vi "SC10_set_mode2.vi"(6 "error in (no error)":errorcluster, 8 "mode":i32(ring)=3 items=["manual"=1, "auto"=2, "single"=3, "repeat"=4, "external gate"=5], 9 "VISA resource name":refnum<visa-resource-name>) -> (0 "error out":errorcluster, 3 "VISA resource name out":refnum<visa-resource-name>)   [LabVIEW 2010]
panel:
  out "substring":string
  out "read buffer":string
  out "return count 3":u32
  out "return count":u32
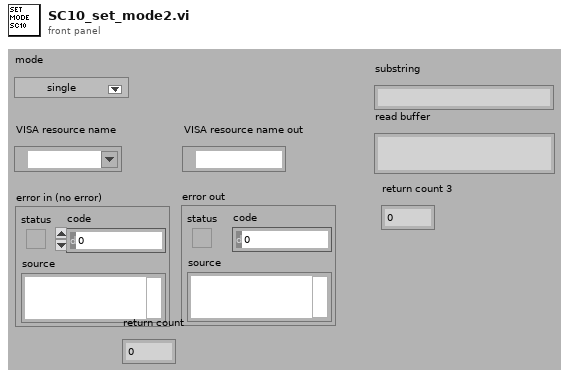
[diagram p1: front panel]
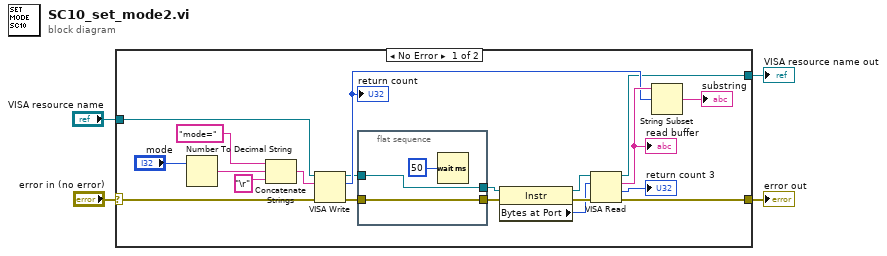
[diagram p0: block diagram]
diagram:
  n1 = case shown="No Error" "error in (no error)" {
    selector: "error in (no error)" -> [w24 w28]
    tunnel: [w6 w28] -> w3
    tunnel: [w5 w29] -> w2
    tunnel: "VISA resource name" -> [w23 w29]
    frame No Error {
      n2 = Number To Decimal String(number="mode") -> (decimal integer string=w19:string)  [unwired: 1 in]
      n3 = Concatenate Strings("mode=" ("string"), w19, "\r" ("write buffer")) -> (w20:string)
      n4 = VISA Write(VISA resource name=w23, write buffer=w20, error in (no error)=w24) -> (VISA resource name out=w8:refnum<visa-resource-name>, return count=w9:u32, error out=w7:errorcluster)
      "return count" <- w9
      n5 = flat-sequence {
        tunnel: w8 -> [w26]
        tunnel: [w26] -> w12
        tunnel: w7 -> [w25]
        tunnel: [w25] -> w13
        frame #0 {
          n6 = Wait (ms)(milliseconds to wait=u32 50) -> ()  [unwired: 1 out]
        }
      }
      n7 = property class="Instr"(reference=w12, error in=w13) -> (reference out=w11:refnum<visa-resource-name>, error out=w14:errorcluster, "Bytes at Port"=w10:u32)
      n8 = VISA Read(VISA resource name=w11, byte count=w10, error in (no error)=w14) -> (VISA resource name out=w5:refnum<visa-resource-name>, read buffer=w16:string, return count=→"return count 3":u32, error out=w6:errorcluster)
      "read buffer" <- w16
      n9 = String Subset(string=w16, offset (0)=w9) -> (substring=→"substring":string)  [unwired: 1 in]
    }
    frame Error {
    }
  }
  "error out" <- w3
  "VISA resource name out" <- w2
